vi "at Max velocity.vi"(8 "error in (no error) 2":errorcluster, 10 "Wanted RPM":dbl) -> (0 "error out 2":errorcluster, 3 "Max Velocity":bool)   [LabVIEW 2017]
panel:
  # "This needs changed with the right Talons stuff"
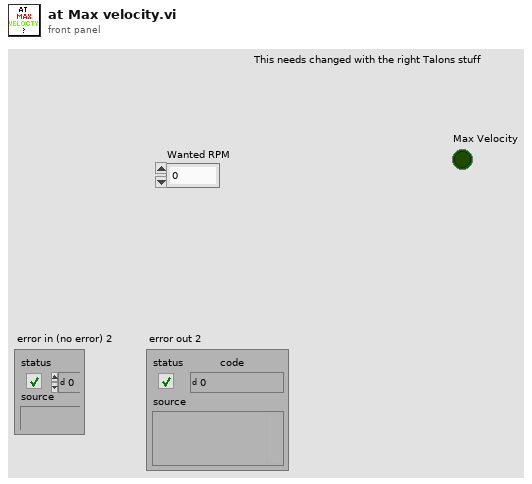
[diagram p1: front panel]
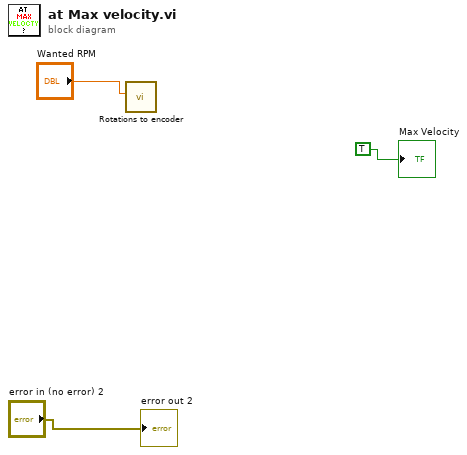
[diagram p0: block diagram]
diagram:
  n1 = call "Rotations to encoder.vi"("Rotations"="Wanted RPM") -> ()  [unwired: 10 in, 1 out]
  "Max Velocity" <- TRUE
  "error out 2" <- "error in (no error) 2"
